vi "Configure Channel Connection.vi"(6 "Break Before Make (OFF)":bool, 7 "Exclusive Close (OFF)":bool, 8 "error in":errorcluster, 11 "VISA resource name":refnum<visa-resource-name>) -> (0 "error out":errorcluster, 3 "VISA resource name out":refnum<visa-resource-name>)   [LabVIEW 2018, in "Keithley 7001.lvlib"]
uses:
  <instrlib>/Keithley 7001/Keithley 7001.lvlib
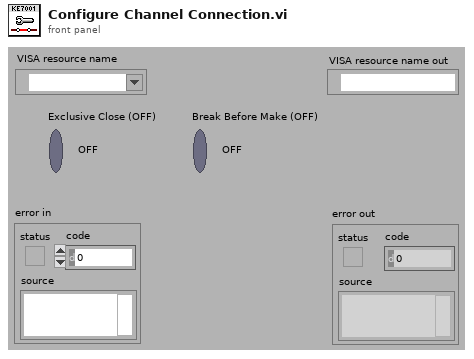
[diagram p1: front panel]
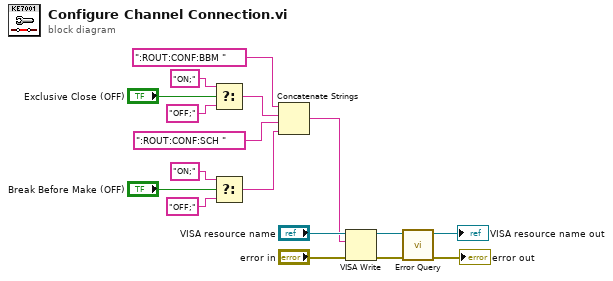
[diagram p0: block diagram]
diagram:
  n1 = Select(t="ON;", s="Exclusive Close (OFF)", f="OFF;") -> (s? t:f=w4:string)
  n2 = Select(t="ON;", s="Break Before Make (OFF)", f="OFF;") -> (s? t:f=w2:string)
  n3 = Concatenate Strings(":ROUT:CONF:BBM ", w4, ":ROUT:CONF:SCH ", w2) -> (w1:string)
  n4 = VISA Write(VISA resource name="VISA resource name", write buffer=w1, error in (no error)="error in") -> (VISA resource name out=w17:refnum<visa-resource-name>, error out=w16:errorcluster)  [unwired: 1 out]
  n5 = call <instrlib>:"Error Query.vi"("error in (no error)"=w16, "VISA resource name"=w17) -> ("error out"=→"error out":errorcluster, "VISA resource name out"=→"VISA resource name out":refnum<visa-resource-name>)  [unwired: 6 in, 2 out]
